vi "day_1.vi"() -> ()   [LabVIEW 2020]
panel:
  out "total":i32
  out "ratio  3":dbl
  out "ratio  4":dbl
  out "ratio  6":dbl
  out "ratio  5":dbl
  out "ratio  2":dbl
  out "ratio":dbl
  out "6":i32
  out "5":i32
  out "4":i32
  out "3":i32
  out "2":i32
  out "1":i32
  out "XY Graph":cluster{dbl[], dbl[]}(graph)
  out "Array":i32[](array[numeric])
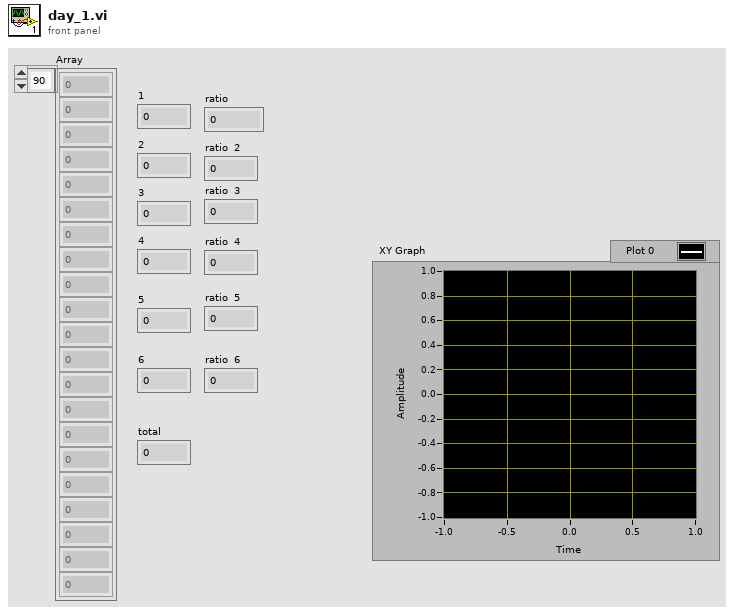
[diagram p1: front panel]
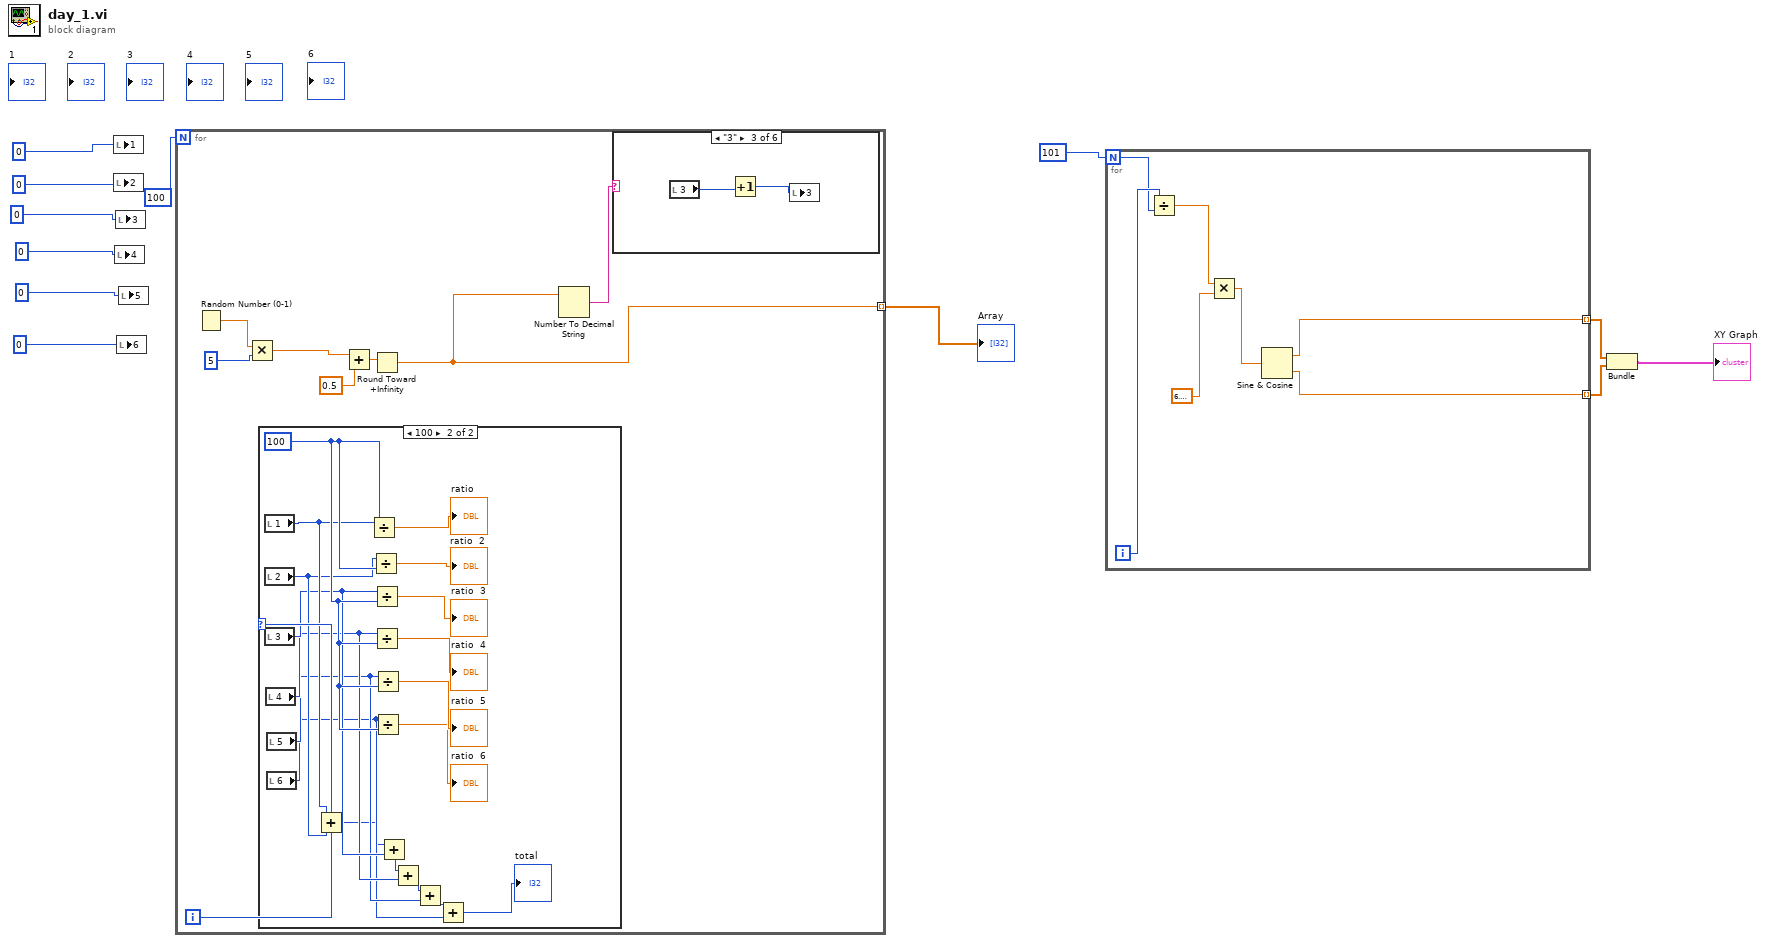
[diagram p0: block diagram]
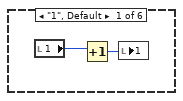
[diagram p2: hidden frame]
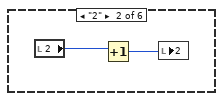
[diagram p3: hidden frame]
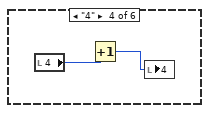
[diagram p4: hidden frame]
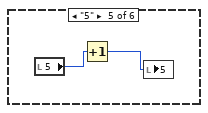
[diagram p5: hidden frame]
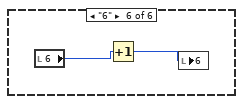
[diagram p6: hidden frame]
diagram:
  n1 = local write "1"(0) -> ()
  n2 = local write "2"(0) -> ()
  n3 = local write "4"(0) -> ()
  n4 = local write "3"(0) -> ()
  n5 = local write "6"(0) -> ()
  n6 = local write "5"(0) -> ()
  n7 = for {
    N: 100 -> [_]
    tunnel: [w15] -> w11 mode=indexing
    i -> [w13]
    n8 = Random Number (0-1)() -> (number: 0 to 1=w19:dbl)
    n9 = Multiply(x=w19, y=5) -> (x*y=w18:dbl)
    n10 = case shown="100" w13 {
      frame 0, Default {
      }
      frame 100 {
        w44 = 100
        n11 = local read "1"() -> (w43:i32)
        n12 = local read "2"() -> (w42:i32)
        n13 = local read "3"() -> (w41:i32)
        n14 = local read "4"() -> (w40:i32)
        n15 = local read "5"() -> (w39:i32)
        n16 = local read "6"() -> (w38:i32)
        n17 = Add(x=w43, y=w42) -> (x+y=w37:i32)
        n18 = Divide(x=w43, y=w44) -> (x/y=→"ratio":dbl)
        n19 = Divide(x=w42, y=w44) -> (x/y=→"ratio  2":dbl)
        n20 = Divide(x=w41, y=w44) -> (x/y=→"ratio  3":dbl)
        n21 = Divide(x=w40, y=w44) -> (x/y=→"ratio  4":dbl)
        n22 = Divide(x=w39, y=w44) -> (x/y=→"ratio  5":dbl)
        n23 = Divide(x=w38, y=w44) -> (x/y=→"ratio  6":dbl)
        n24 = Add(x=w37, y=w41) -> (x+y=w36:i32)
        n25 = Add(x=w36, y=w40) -> (x+y=w35:i32)
        n26 = Add(x=w35, y=w39) -> (x+y=w34:i32)
        n27 = Add(x=w34, y=w38) -> (x+y=→"total":i32)
      }
    }
    n28 = Add(x=w18, y=0.5) -> (x+y=w16:dbl)
    n29 = Round Toward +Infinity(x=w16) -> (ceil(x): smallest int >= x=w15:dbl)
    n30 = Number To Decimal String(number=w15) -> (decimal integer string=w14:string)  [unwired: 1 in]
    n31 = case shown="\"3\"" w14 {
      frame "1", Default {
        n32 = local read "1"() -> (w22:i32)
        n33 = Increment(x=w22) -> (x+1=w21:i32)
        n34 = local write "1"(w21) -> ()
      }
      frame "2" {
        n35 = local read "2"() -> (w24:i32)
        n36 = Increment(x=w24) -> (x+1=w23:i32)
        n37 = local write "2"(w23) -> ()
      }
      frame "3" {
        n38 = local read "3"() -> (w26:i32)
        n39 = Increment(x=w26) -> (x+1=w25:i32)
        n40 = local write "3"(w25) -> ()
      }
      frame "4" {
        n41 = local read "4"() -> (w28:i32)
        n42 = Increment(x=w28) -> (x+1=w27:i32)
        n43 = local write "4"(w27) -> ()
      }
      frame "5" {
        n44 = local read "5"() -> (w30:i32)
        n45 = Increment(x=w30) -> (x+1=w29:i32)
        n46 = local write "5"(w29) -> ()
      }
      frame "6" {
        n47 = local read "6"() -> (w32:i32)
        n48 = Increment(x=w32) -> (x+1=w31:i32)
        n49 = local write "6"(w31) -> ()
      }
    }
  }
  "Array" <- w11
  n50 = for {
    N: 101 -> [w51]
    tunnel: [w54] -> w10 mode=indexing
    tunnel: [w53] -> w9 mode=indexing
    i -> [w52]
    n51 = Divide(x=w52, y=w51) -> (x/y=w57:dbl)
    n52 = Multiply(x=w57, y=6.283185307179586) -> (x*y=w55:dbl)
    n53 = Sine & Cosine(0:w55) -> (1:w54:dbl, 2:w53:dbl)
  }
  n54 = Bundle(w10, w9) -> (→"XY Graph":cluster{dbl[], dbl[]})  [unwired: 1 in]
